vi "CMD_MPGON.vi"(6 "Gantry in":refnum<class "Gantry.lvclass">, 8 "error in (no error)":errorcluster, 10 "Arguments":string[](array[string]), 11 "gScript Interpreter in":refnum<class "gScript Interpreter.lvclass">) -> (0 "error out":errorcluster, 3 "gScript Interpreter out":refnum<class "gScript Interpreter.lvclass">, 4 "Gantry out":refnum<class "Gantry.lvclass">)   [LabVIEW 2017, in "gScript Interpreter.lvclass"]
uses:
  gScript Interpreter.lvclass
  Shared Components/Gantry Class/Gantry.lvclass
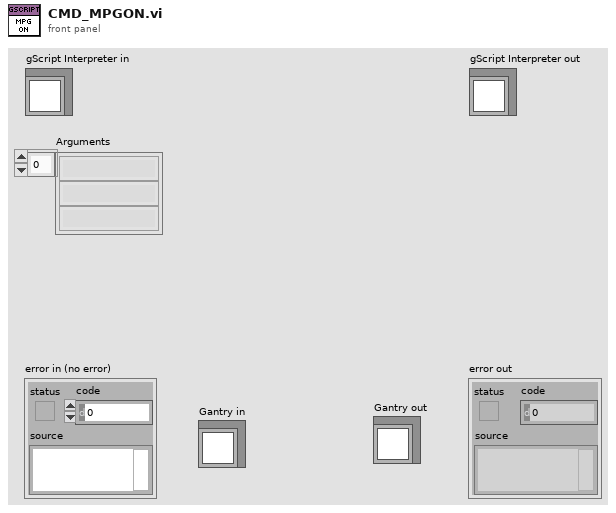
[diagram p1: front panel]
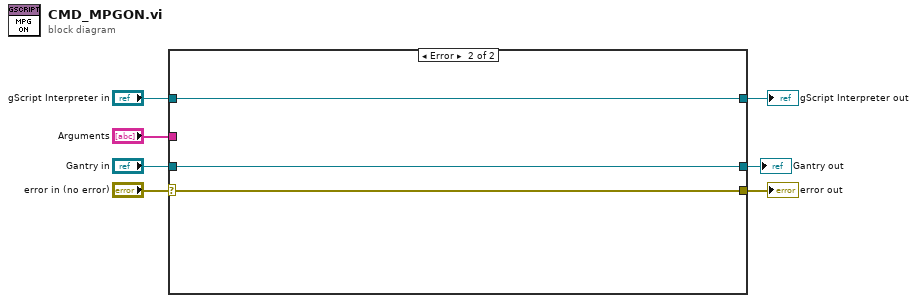
[diagram p0: block diagram]
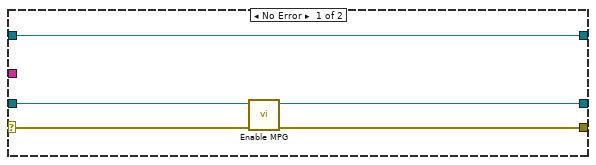
[diagram p2: hidden frame]
diagram:
  n1 = case shown="Error" "error in (no error)" {
    selector: "error in (no error)" -> [w10 w15]
    tunnel: [w9 w15] -> w6
    tunnel: [w8 w14] -> w4
    tunnel: "gScript Interpreter in" -> [w8 w14]
    tunnel: "Arguments" -> [_ _]
    tunnel: "Gantry in" -> [w12 w13]
    tunnel: [w11 w13] -> w1
    frame No Error {
      n2 = call-dynamic "Enable MPG.vi"("error in"=w10, "Gantry in"=w12) -> ("error out"=w9:errorcluster, "Gantry out"=w11:refnum<class "Gantry.lvclass">)  [unwired: 8 in]
    }
    frame Error {
    }
  }
  "error out" <- w6
  "gScript Interpreter out" <- w4
  "Gantry out" <- w1
